vi "Cam2.vi"() -> ()   [LabVIEW 2018]
panel:
  out "等待时间":i32
  out "发散角":cluster{"横向发散角":dbl, "纵向发散角":dbl}
  out "远场光斑中心":cluster{"X Centroid":sgl, "Y Centroid":sgl} {"Y Centroid" format="%.2f"; "X Centroid" format="%.2f"}
  out "近场光斑中心":cluster{"X Centroid":sgl, "Y Centroid":sgl} {"Y Centroid" format="%.2f"; "X Centroid" format="%.2f"}
  out "状态提示":string
  out "当前曝光us":dbl
  out "近场图":T1(plugin-control)
  in  "重新连接相机":bool
  in  "采集":bool
  in  "数据输出":i32[](listbox)
  out "通信":bool
  out "远场图":T1(plugin-control)
  out "error out":errorcluster caption="error in (no error)"
  in  "error in (no error)":errorcluster
  in  "触发方式":enum8{"软件触发", "上升沿触发", "下降沿触发"}(ring)
  in  "曝光设置 us":dbl=100.0 min=100.0 max=2000000.0 format="%#.1f"
  # "确认参数后点击”近场采集“按钮进行测量"
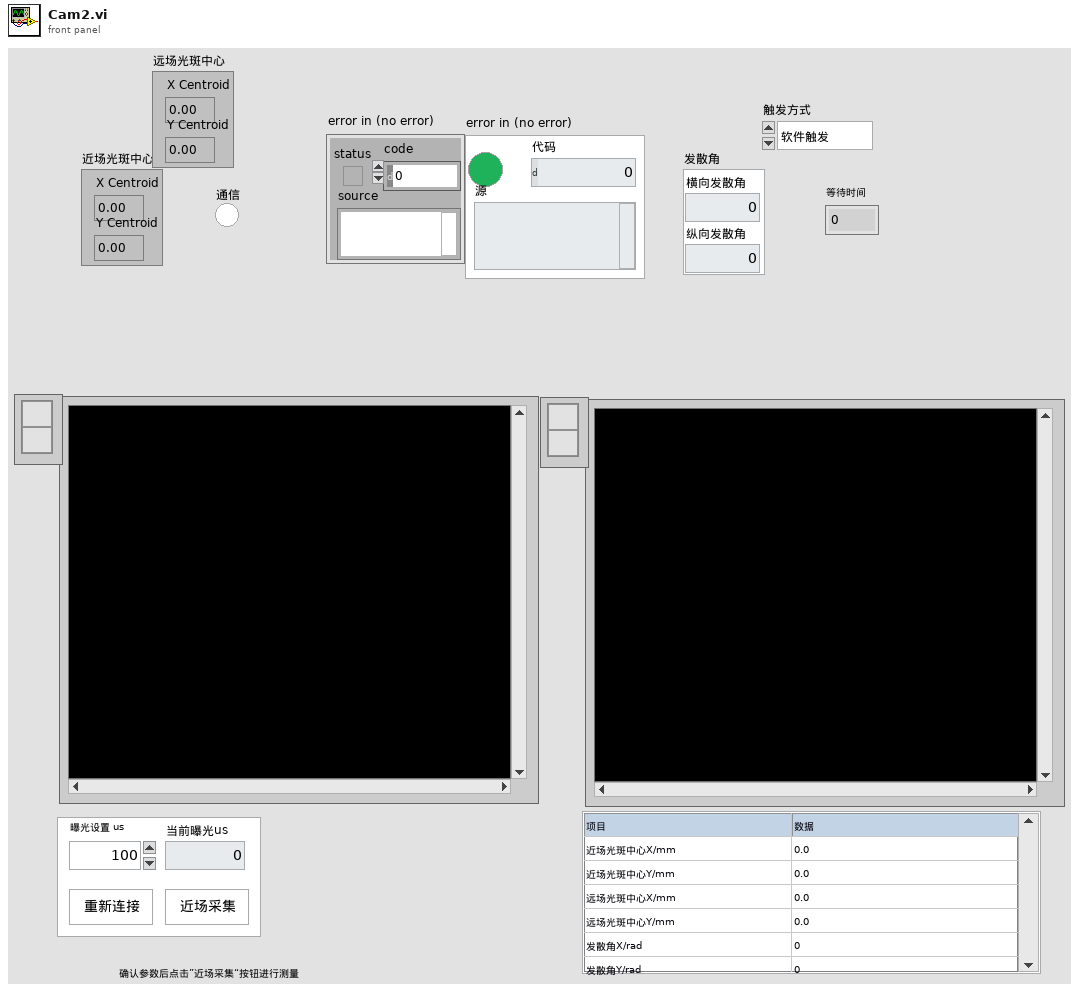
[diagram p1: front panel]
types:
  T1 = typedef "IMAQ Image.ctl" = refnum<image>
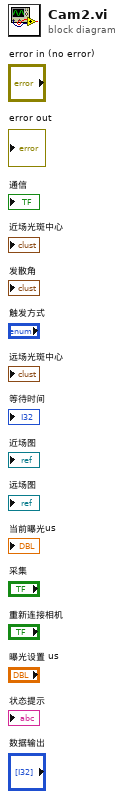
[diagram p0: block diagram]
diagram:
